vi "WrapTime.vi"(11 "SetTime":u32=750) -> (3 "TimesUP":bool)   [LabVIEW 2011]
uses:
  Robot Global Data.vi
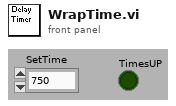
[diagram p1: front panel]
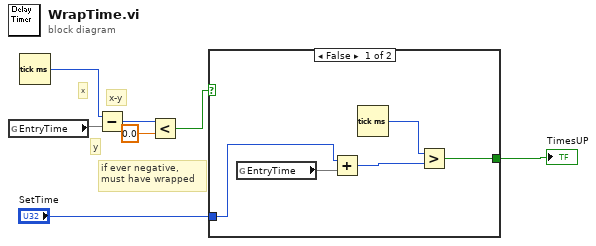
[diagram p0: block diagram]
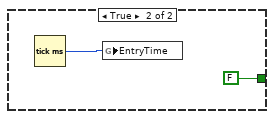
[diagram p2: hidden frame]
diagram:
  # "x-y"
  # "y"
  # "x"
  # "if ever negative, \nmust have wrapped"
  n1 = global read "Robot Global Data.vi" "EntryTime"() -> (w3)
  n2 = Tick Count (ms)() -> (millisecond timer value=w7:u32)
  n3 = Subtract(x=w7, y=w3) -> (x-y=w6:u32)
  n4 = Less?(x=w6, y=0.0) -> (x < y?=w4:bool)
  n5 = case shown="False" w4 {
    tunnel: [w9 FALSE] -> w2
    tunnel: "SetTime" -> [w8 _]
    frame False {
      n6 = global read "Robot Global Data.vi" "EntryTime"() -> (w12)
      n7 = Add(x=w8, y=w12) -> (x+y=w11:u32)
      n8 = Tick Count (ms)() -> (millisecond timer value=w10:u32)
      n9 = Greater?(x=w10, y=w11) -> (0:w9:bool)
    }
    frame True {
      n10 = Tick Count (ms)() -> (millisecond timer value=w14:u32)
      n11 = global write "Robot Global Data.vi" "EntryTime"(w14) -> ()
    }
  }
  "TimesUP" <- w2
